vi "Read TagVarNames.vi"(8 "error in (no error)":errorcluster, 11 "Tag Expr in":refnum<class "Tag Expr.lvclass">) -> (0 "error out":errorcluster, 2 "TagVarNames":string[](array[string]), 3 "Tag Expr out":refnum<class "Tag Expr.lvclass">)   [LabVIEW 2020, in "Tag Expr.lvclass"]
uses:
  Tag Expr.lvclass
  Tag Expr.lvclass/Tag Expr.ctl
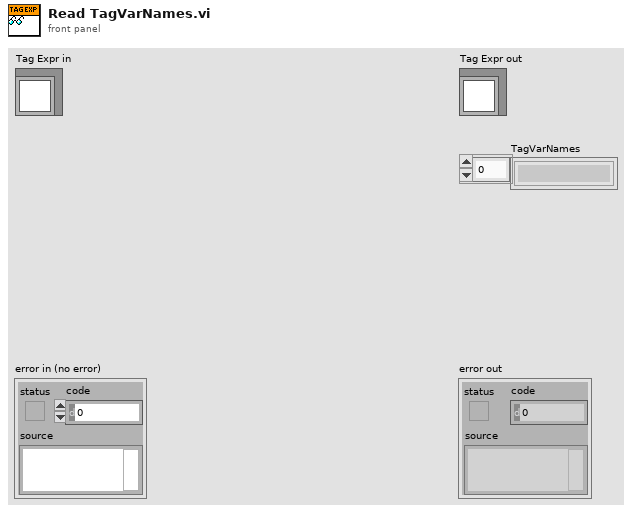
[diagram p1: front panel]
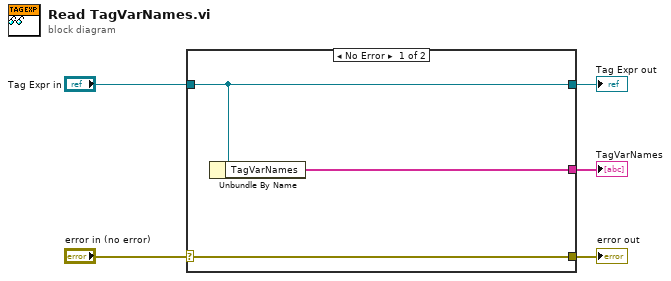
[diagram p0: block diagram]
diagram:
  n1 = case shown="No Error" "error in (no error)" {
    selector: "error in (no error)" -> [w8 w9]
    tunnel: [w8 w9] -> w4
    tunnel: [w7 w10] -> w2
    tunnel: "Tag Expr in" -> [w7 w10]
    tunnel: [w6 _] -> w1
    frame No Error {
      n2 = Unbundle By Name(w7) -> ("TagVarNames"=w6:string[])
    }
    frame Error {
    }
  }
  "error out" <- w4
  "Tag Expr out" <- w2
  "TagVarNames" <- w1
